vi "Read Autonomous Data.vi"(11 "name or relative path":string) -> (3 "transposed array":dbl[][](array[numeric]))   [LabVIEW 2017]
uses:
  <vilib>/Utility/file.llb/Read Delimited Spreadsheet (DBL).vi
panel:
  out "path 2":path
  out "path":path
  out "all rows":dbl[][](array[numeric])
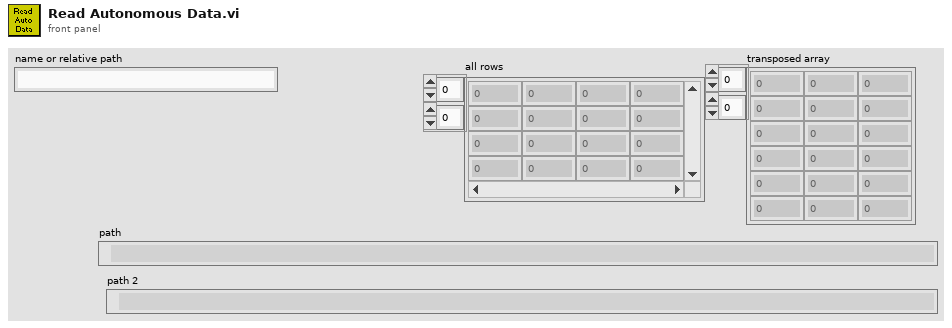
[diagram p1: front panel]
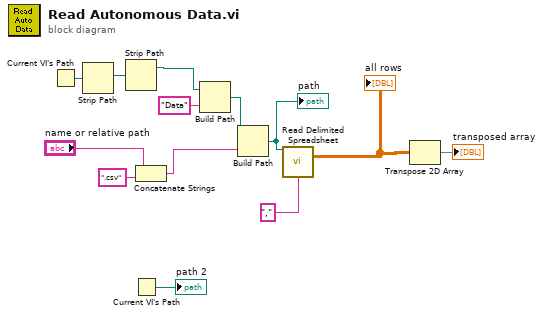
[diagram p0: block diagram]
diagram:
  n1 = Current VI's Path() -> (path=w6:path)
  n2 = Strip Path(path=w6) -> (stripped path=w12:path)  [unwired: 1 out]
  n3 = Strip Path(path=w12) -> (stripped path=w11:path)  [unwired: 1 out]
  n4 = Current VI's Path() -> (path=→"path 2":path)
  n5 = Concatenate Strings("name or relative path", ".csv" ("string")) -> (w9:string)
  n6 = Build Path(base path=w11, name or relative path="Data") -> (appended path=w10:path)
  n7 = Build Path(base path=w10, name or relative path=w9) -> (appended path=w3:path)
  "path" <- w3
  n8 = call-poly <vilib>:"Read Delimited Spreadsheet.vi"("file path (dialog if empty)"=w3, "delimiter (\\t)"="," ("delimiter (\\t)")) -> ("all rows"=w8:dbl[][])  [unwired: 8 in, 5 out]
  "all rows" <- w8
  n9 = Transpose 2D Array(2D array=w8) -> (transposed array=→"transposed array":dbl[][])
